vi "Scan_FileList.vi"(10 "Data Feed":string, 11 "DataCluster":T1) -> (0 "Downloaded bytes":i32, 2 "state out":string, 3 "Sorted Files":string[][](array[string]))   [LabVIEW 2022 SP3]
uses:
  DataCluster.ctl
  bf192da2-a038-4d3f-ab57-7c4c3700bcdc.vi
  <vilib>/Array/Sort 2D Array - Pop Stack.vi
  <vilib>/Array/Sort 2D Array - Push Stack.vi
panel:
  out "substring before match":string
  out "Array":string[][](array[string])
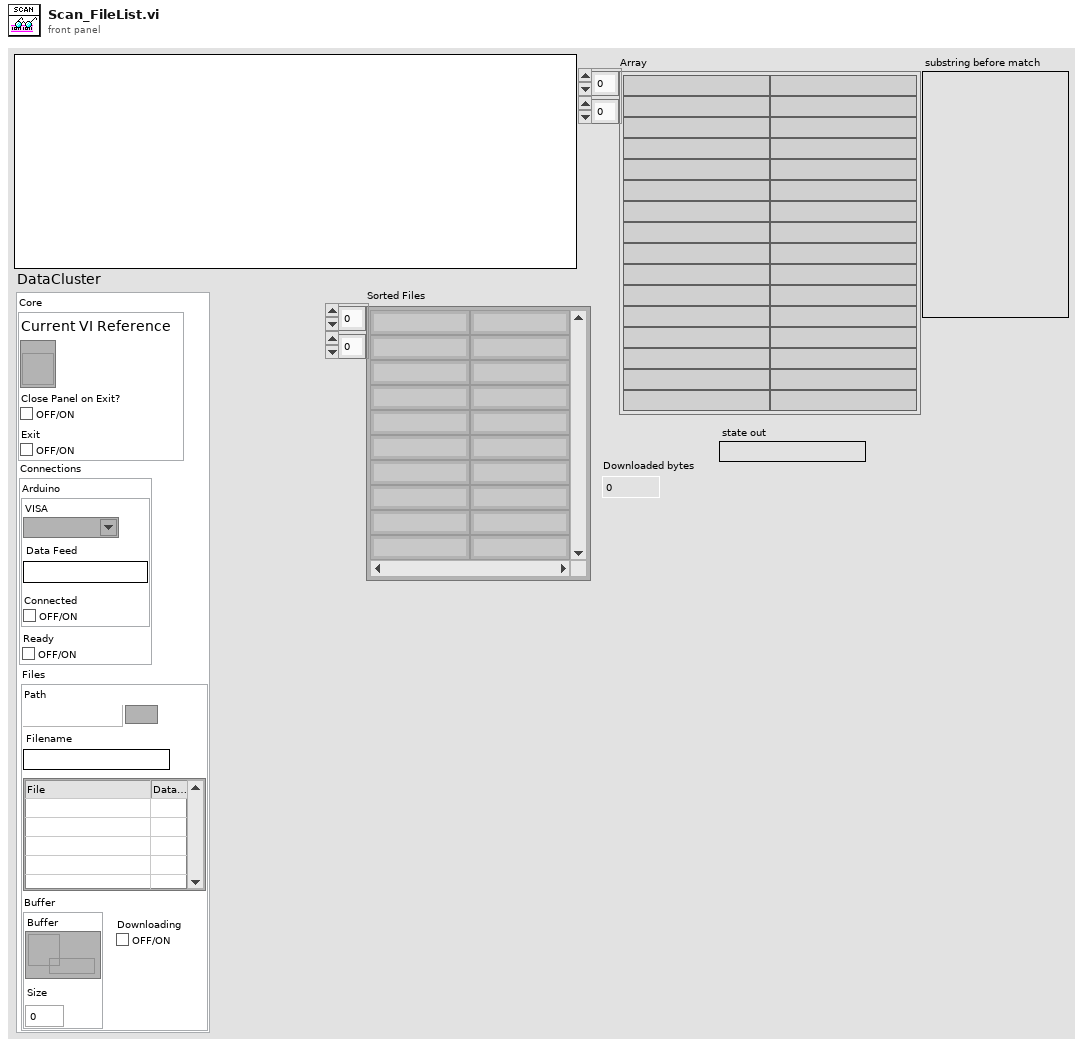
[diagram p1: front panel]
types:
  T1 = typedef "DataCluster.ctl" = cluster{"Core":cluster{"Current VI Reference":refnum<vi>, "Close Panel on Exit?":bool, "Exit":bool}, "Connections":cluster{"Arduino":cluster{"VISA":refnum<visa-resource-name>, "Data Feed":string, "Connected":bool}, "Ready":bool}, "Files":cluster{"Path":path, "Filename":string, "File List":i32, "Buffer":cluster{"Buffer":refnum<queue>, "Size":i32}, "Downloading":bool}}
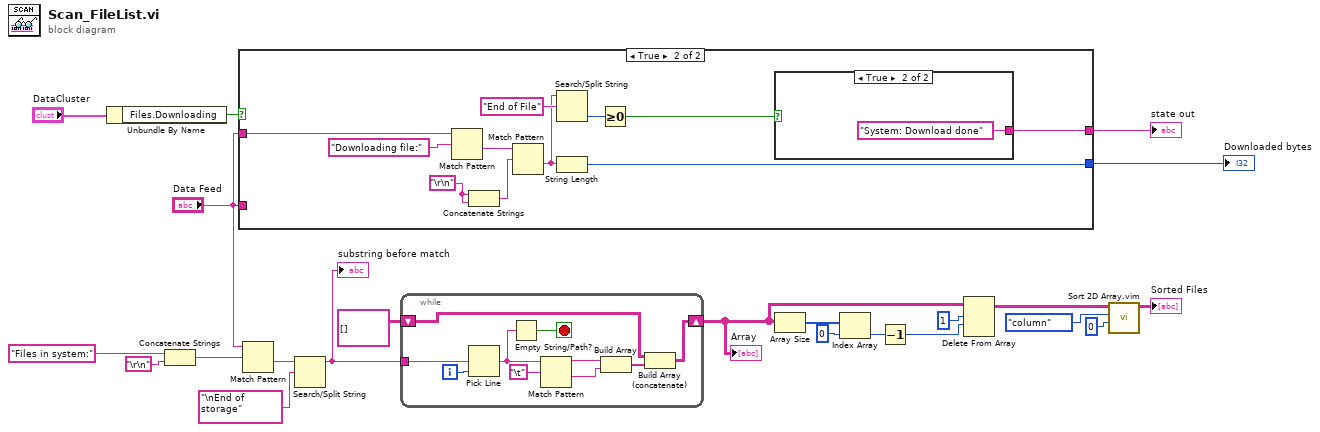
[diagram p0: block diagram]
diagram:
  n1 = Unbundle By Name("DataCluster") -> ("Files.Downloading"=w5:bool)
  n2 = Concatenate Strings("Files in system:" ("search string/char (-)"), "\r\n") -> (w21:string)
  n3 = case shown="True" w5 {
    tunnel: "Data Feed" -> [_ _]
    tunnel: [_ w30] -> w1
    tunnel: "Data Feed" -> [_ w27]
    tunnel: [_ w25] -> w3
    frame False {
    }
    frame True {
      w28 = "\r\n"
      n4 = Match Pattern(string=w27, regular expression="Downloading file:") -> (after substring=w24:string)  [unwired: 1 in, 3 out]
      n5 = Concatenate Strings(w28, w28) -> (w29:string)
      n6 = Match Pattern(string=w24, regular expression=w29) -> (after substring=w23:string)  [unwired: 1 in, 3 out]
      n7 = Search/Split String(string=w23, search string/char (-)="End of File") -> (offset of match=w32:i32)  [unwired: 1 in, 2 out]
      n8 = String Length(string=w23) -> (length=w25:i32)
      n9 = Greater Or Equal To 0?(x=w32) -> (x >= 0?=w31:bool)
      n10 = case shown="True" w31 {
        tunnel: [_ "System: Download done"] -> w30
        frame False {
        }
        frame True {
        }
      }
    }
  }
  "state out" <- w1
  "Downloaded bytes" <- w3
  n11 = Match Pattern(string="Data Feed", regular expression=w21) -> (after substring=w20:string)  [unwired: 1 in, 3 out]
  n12 = Search/Split String(string=w20, search string/char (-)="\nEnd of storage") -> (substring before match=w18:string)  [unwired: 1 in, 2 out]
  "substring before match" <- w18
  n13 = while {
    tunnel: w18 -> [w44]
    shift-right: [w37] -> w10
    shift-left: string[][] [] -> [w36]
    i -> [w43]
    stop <- w42 stop-if-true
    n14 = Pick Line(multi-line string=w44, line index=w43) -> (output string=w41:string)  [unwired: 1 in]
    n15 = Empty String/Path?(string/path=w41) -> (empty?=w42:bool)
    n16 = Match Pattern(string=w41, regular expression="\t") -> (before substring=w40:string, after substring=w39:string)  [unwired: 1 in, 2 out]
    n17 = Build Array(w40, w39) -> (w38:string[])
    n18 = Build Array (concatenate)(w36, w38) -> (w37:string[][])
  }
  "Array" <- w10
  n19 = Array Size(array=w10) -> (size(s)=w15:i32[])
  n20 = Index Array(array=w15, index=0) -> (element=w13:i32)
  n21 = Decrement(x=w13) -> (x-1=w11:i32)
  n22 = Delete From Array(array=w10, length=1, index (row)=w11) -> (array with subset deleted=w7:string[][])  [unwired: 1 in, 1 out]
  n23 = call "Sort 2D Array.vim"("index"=0, "dimension to index (column)"=enum16{"column", "row"}."column", "2D array"=w7) -> ("sorted 2D array"=→"Sorted Files":string[][])  [unwired: 7 in, 1 out]
